vi "Merge Errors - Conditional.vi"(7 "error to merge":errorcluster, 10 "upstream error":errorcluster, 11 "error?":bool) -> (2 "merged error":errorcluster)   [LabVIEW 2018, in "Utilities.lvlib"]
uses:
  Utilities.lvlib
panel:
  # "Connector Pane"
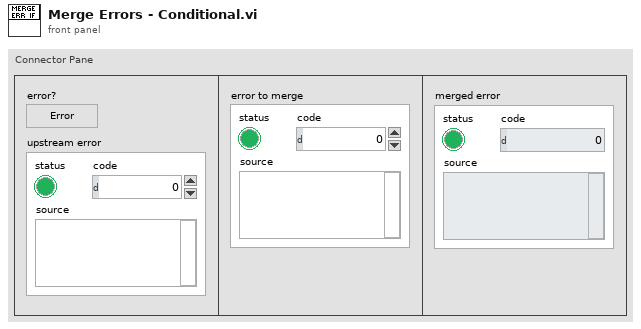
[diagram p1: front panel]
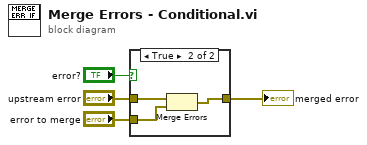
[diagram p0: block diagram]
diagram:
  n1 = case shown="True" "error?" {
    tunnel: "upstream error" -> [w5 w8]
    tunnel: [w5 w7] -> w3
    tunnel: "error to merge" -> [_ w6]
    frame False {
    }
    frame True {
      n2 = Merge Errors(w8, w6) -> (w7:errorcluster)
    }
  }
  "merged error" <- w3
